vi "Load App.vi"(8 "error in (no error)":errorcluster, 11 "Controller Actor.lvlib:Controller.lvclass":refnum<class "Controller.lvclass">) -> (0 "error out":errorcluster)   [LabVIEW 2026, in "Controller Actor.lvlib" / "Controller.lvclass"]
uses:
  Controller.lvclass
  Controller.lvclass/Controller.ctl
  <vilib>/ActorFramework/Actor/Actor.lvclass
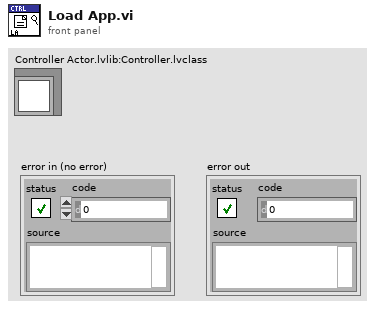
[diagram p1: front panel]
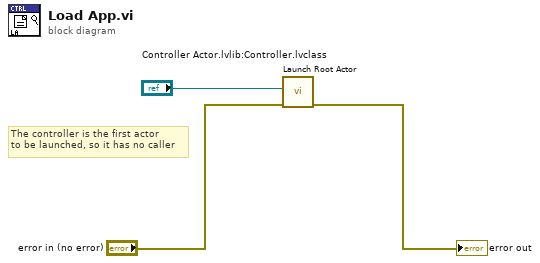
[diagram p0: block diagram]
diagram:
  # "The controller is the first actor\nto be launched, so it has no caller"
  n1 = call <vilib>:"Launch Root Actor.vi"("error in (no error)"="error in (no error)", "Actor"="Controller Actor.lvlib:Controller.lvclass") -> ("error out"=→"error out":errorcluster)  [unwired: 8 in, 1 out]
